vi "TestCounter.Increment.vi"(8 "error in":errorcluster) -> (0 "error out":errorcluster, 1 "TestCount after":u64, 2 "TestCount before":u64, 5 "TestCount path":path)   [LabVIEW 2019, in "Tools.lvlib"]
uses:
  Tools.lvlib
  ProjectPaths.ctl
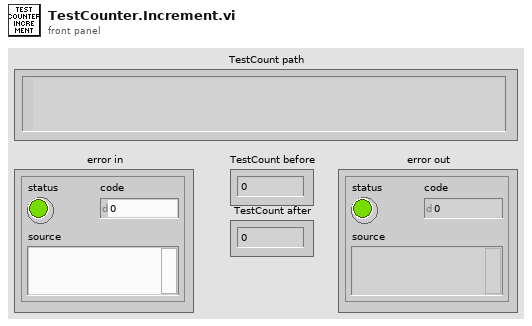
[diagram p1: front panel]
types:
  T1 = typedef "Tools.lvlib/ProjectPaths.ctl" = enum16{"Settings dir", "Logs dir", "Resources dir", "Verification file", "Users file", "Root dir"}
  T2 = enum16{"open", "replace", "create", "open or create", "replace or create", "replace or create with confirmation"}
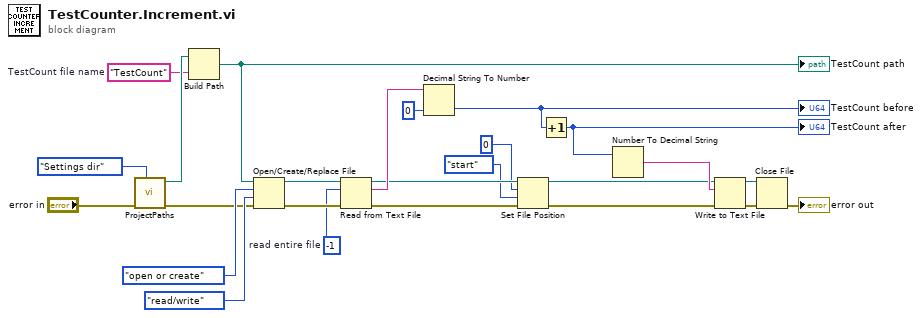
[diagram p0: block diagram]
diagram:
  w16 = -1  # read entire file
  w22 = "TestCount"  # TestCount file name
  n1 = call "ProjectPaths.vi"("Item"=ProjectPaths."Settings dir", "Error In"="error in") -> ("Error Out"=w18:errorcluster, "Path"=w23:path)  [unwired: 8 in]
  n2 = Build Path(base path=w23, name or relative path=w22) -> (appended path=w21:path)
  "TestCount path" <- w21
  n3 = Open/Create/Replace File(file path (use dialog)=w21, error in=w18, operation (0:open)=T2."open or create", access (0:read/write)=enum16{"read/write", "read-only", "write-only"}."read/write") -> (refnum out=w25:refnum<file>, error out=w24:errorcluster)  [unwired: 2 in, 1 out]
  n4 = Read from Text File(file (use dialog)=w25, count=w16, error in=w24) -> (refnum out=w5:refnum<file>, text=w15:string, error out=w7:errorcluster)  [unwired: 1 in, 1 out]
  n5 = Decimal String To Number(string=w15, default (0L)=u64 0 ("default (0 I32)")) -> (number=w13:u64)  [unwired: 1 in, 1 out]
  "TestCount before" <- w13
  n6 = Set File Position(offset (in bytes) (0)=i64 0, refnum=w5, from (0:start)=enum16{"start", "end", "current"}."start", error in=w7) -> (refnum out=w4:refnum<file>, error out=w6:errorcluster)
  n7 = Increment(x=w13) -> (x+1=w10:u64)
  "TestCount after" <- w10
  n8 = Number To Decimal String(number=w10) -> (decimal integer string=w8:string)  [unwired: 1 in]
  n9 = Write to Text File(file (use dialog)=w4, text=w8, error in=w6) -> (refnum out=w12:refnum<file>, error out=w11:errorcluster)  [unwired: 1 in, 1 out]
  n10 = Close File(refnum=w12, error in=w11) -> (error out=→"error out":errorcluster)  [unwired: 1 out]
